vi "FestoCPX.Station.LaserPress.Ready.vi"(7 "Log (T)":bool=TRUE, 8 "error in":errorcluster, 10 "Position":T2) -> (0 "error out":errorcluster, 2 "Ready state":T1)   [LabVIEW 2015]
uses:
  tools/Translator/Translator.Message.ctl
  tools/EventLog/EventLog.EventSource.ctl
  FestoCPX.Station.LaserPress.ReadyState.ctl
  tools/EventLog/EventLog.CreateError(array).vi
  Station/Station.ValvePosition.ctl
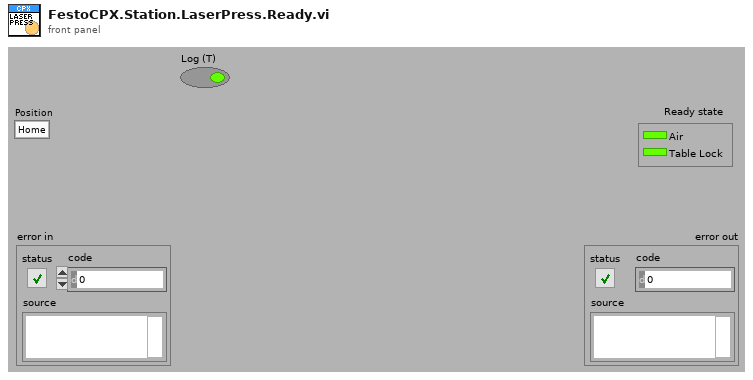
[diagram p1: front panel]
types:
  T1 = typedef "FestoCPX.Station.LaserPress.ReadyState.ctl" = cluster{"Air":bool, "Table Lock":bool}
  T2 = typedef "Station.ValvePosition.ctl" = enum16{"Home", "Work"}
  T3 = typedef "EventLog.EventSource.ctl" = enum16{"All", "Gui", "Ref", "File", "Seq", "Scan", "Lock", "AO", "AI", "CI", "DIO", "CPX", "PS", "Proda", "Trace", "Laser", "Keyence"}
  T4 = typedef "Translator.Message.ctl" = enum16{"-", "Event confirmed", "Log out", "Log in", "Shutdown", "Cancel", "Start", "On", "Off", "OK", "NOK", "NOK %s", "Home", "Work", "In progress...", "Missing", "Empty", "Hardware failure", "Initial", "Error %d >> %s", "Error %d >> %s >> %s", "Msg %d >> %s", "Unable to reset Laser Interlock", "Unable to reset Laser Shutterlock. Laser not ready", "Starting %s", "Quitting %s", "Configured", "Initializing", "Quitting", "Loading", "Running", "Stopped", "Summary", "Laser", "Do you want to continue?", "Station is not based. Do you want to exit?", "Station requires changeover. Do you want to run the test?", "Test options are not set as default. Do you want to continue?", "Connect ATEQ to terminal and set leakage to 0", "Set no leakage at ATEQ", "Set desired leakage at ATEQ at terminal M1 or skip", "Set desired leakage at ATEQ at terminal M3/M21/M22 or skip", "Set desired leakage at ATEQ at terminal M12 or skip", "Set desired leakage at ATEQ at terminal M1/M3 or skip", "Set desired leakage at ATEQ at terminal M21/M22 or skip", "Set desired leakage at ATEQ at terminal M1/M21/M22 or skip", "Calibration", "Log out?", "System", "All", "IDLE", "Translating...%s", "Not found", "Alarm %s", "Run", "Skip", "Abort", "Repeat", "Please wait...", "Database disconnected", "Database disconnected - changeover disabled!", "Login to database successful", "Login to database failed: %d; %s", "Unable to check the product status of reference %d - database disconnected", "Unable to set the product status of reference %d - database disconnected", "Variant file backup %s", "Read steps (%s)", "Result", "Station armed!", "Station requires changeover!", "Select reference number...", "EMERGENCY CURTAIN", "EMERGENCY BUTTON - press Control button", "EMERGENCY DOOR - press Control button", "Unable to reset safety circuit - Emergency Button pressed", "Unable to reset safety circuit - Emergency Doors open", "Station not based", "Station basing...", "Unkown reference", "Reference %d missing", "Test %s", "Test OK", "Test NOK", "Test NOK - press Confirm button", "Test error - press Confirm button", "Test stopped", "Station ready / Prepare product", "Station ready / Press start to scan product", "Station ready / Scanning product", "Rotating table...", "Rotating table... on hold by curtain", "Table rotated in %.1f seconds", "Table rotation aborted - Emergency button", "Table rotation aborted - Emergency door", "Table rotation aborted - Air pressure 1 off", "Table rotation aborted - Air pressure 2 off", "Test running... / Prepare next product", "Test running... / Press start to scan next product", "Test running... / Scanning next product...", "Test running... / Next products will start automatically", "Test running... / Scanning failed", "Stopping test...", "Finalizing test...", "Sequence folder '%s' is missing", "File '%s' is missing", "File '%s' is broken", "File '%s' is running", "Log file '%s' started", "Step '%s' added to log file", "Step '%s' graph added to log file", "Log file '%s' ended", "Log file '%s' ignored", "Log file '%s' exported", "Log file '%s' export failed", "Wrong serial number in log file", "Test steps are missing", "Output %s = %.3f", "Unable to output %s = %.1f (FB = %.1f; SP = %.1f)", "Unable to stabilize %s = %.1f (SP = %.1f)", "Assembly timeout", "Disassembly timeout", "Assembly %d | %25s | %.02f | %d", "Disassembly %d | %25s | %.02f | %d", "Process param '%s' not found in DB", "Process param '%s' wrong order", "Process param '%s' value %.3f out of limits (%.3f; %.3f)", "Step%d param '%s' not found in DB", "Step%d param '%s' wrong order", "Step%d param '%s' value %.3f out of limits (%.3f; %.3f)", "Step%d EV '%s' not found in DB", "Step%d EV '%s' wrong order", "Reference %d accepted", "Sequence started", "Sequence done", "Sequence aborted at step %d", "Sequence aborted at work", "Sequence aborted at home", "Sequence stopped at step %d", "Sequence error at step %d", "Seqeunce error at home", "Sequence error at work", "Scan plate failed", "Scan laser failed", "Scan plate failed. Error %s", "Scan laser failed. Error %s", "Scan plate failed. Scanner disconnected", "Scan laser failed. Scanner disconnected", "Scan plate failed. Wrong reference %d (expected %d)", "Scan plate failed. Serial number %d/%d did not pass the previous station (status %d)", "Scan plate OK %d/%d", "Scan laser OK", "Scan plate failed. Code missing", "Scan laser failed. Code missing", "Plate scanner OK", "Plate scanner failed. Press confirm button", "Scanning plate...", "%s = %d", "%s = %d->%d", "Motor initialized", "Motor homing", "Motor homed", "Motor home timeout", "Motor home failure. Unable to reset encoder counter (motor pos %.2f; enc pos %.2f)", "Motor started @ %.2f (%s; %.2f; %.1f)", "Motor updated @ %.2f (%s; %.2f; %.1f)", "Motor stopped @ %.2f", "Motor stop timeout", "Motor reached the position @ %.2f", "Motor reached the torque @ %.2f; %.2f", "Motor reached the pressure @ %.2f; %.2f", "Motor timeout (sp %.2f; pv %.2f)", "Unable to move motor - Forks not in Home position", "Screwdriver start timeout", "Screwdriver stop timeout", "Not homed", "Leak test timeout", "Unable to set %s = %.2f - air pressure off", "Unable to reset Emergency Circuit - emg button", "Unable to reset Emergency Circuit - light curtain", "Unable to reset Emergency Circuit - door open", "Unable to set digital output '%s' = %d", "Unable to switch on Air Main Valve - timeout", "Unable to switch off Air Main Valve - timeout", "Unable to rotate Table - timeout", "Unable to rotate Table - air pressure off", "Unable to rotate Table - Press not in Home position", "Unable to rotate Table - Pneumatic & Electric Conn not in Home position", "Unable to rotate Table - Exhaust Conn not in Home position", "Unable to rotate Table - unlock before movement timeout", "Unable to rotate Table - lock after movement timeout", "Unable to move Table Lock to %s position - timeout", "Unable to move Table Lock to %s position - air pressure off", "Unable to move Table Lock to %s position - Table not in position", "Unable to move Product Press to %s position - timeout", "Unable to move Product Press to %s position - air pressure off", "Unable to move Product Press to %s position - Table not locked", "Unable to move Product Press to %s position - Pneumatic & Electric Conn not in Home position", "Unable to move Product Press to %s position - Exhaust Conn not in Home position", "Unable to move Pneumatic & Electric Conn to %s position - timeout", "Unable to move Pneumatic & Electric Conn to %s position - air pressure off", "Unable to move Pneumatic & Electric Conn to %s position - Product Press not in Work position", "Unable to move Vent %s to %s position - timeout", "Unable to move Vent %s to %s position - air pressure off", "Unable to move Vent %s to %s position - Product Press not in Work position", "Unable to move Laser Press to %s position - timeout", "Unable to move Laser Press to %s position - air pressure off", "Unable to move Laser Press to %s position - Table not locked"}
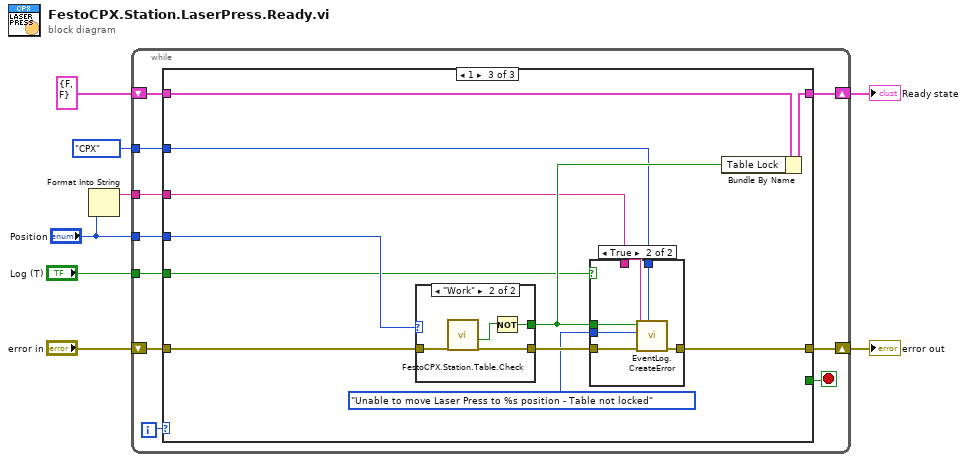
[diagram p0: block diagram]
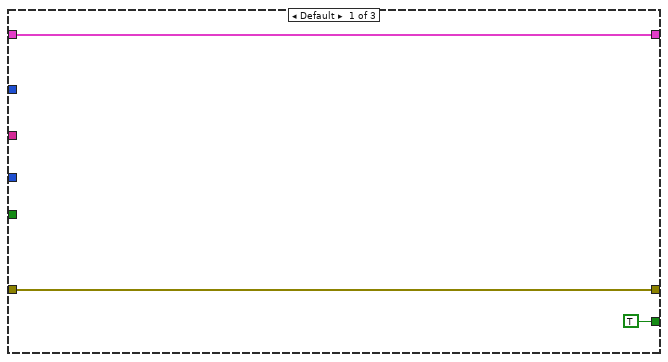
[diagram p2: hidden frame]
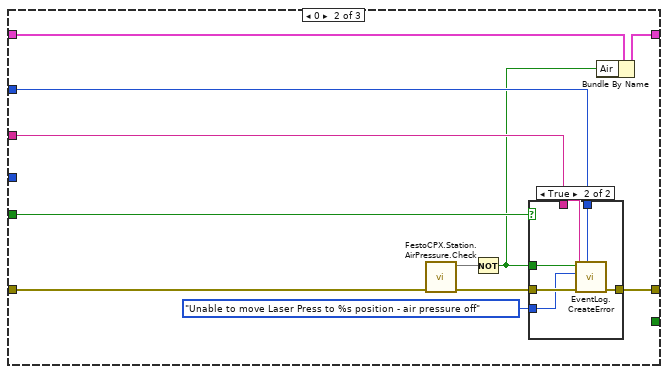
[diagram p3: hidden frame]
diagram:
  n1 = Format Into String("Position") -> (resulting string=w2:string)  [unwired: 3 in, 1 out]
  n2 = while {
    tunnel: "Log (T)" -> [w17]
    tunnel: w2 -> [w16]
    tunnel: EventLog.EventSource."CPX" ("Source") -> [w15]
    shift-right: [w10] -> w5
    shift-left: "error in" -> [w18]
    shift-right: [w11] -> w3
    shift-left: T1 {"Air"=FALSE, "Table Lock"=FALSE} ("Ready state") -> [w12]
    tunnel: "Position" -> [w9]
    i -> [w14]
    stop <- w13 stop-if-true
    n3 = case shown="1" w14 {
      tunnel: w18 -> [w20 w23 w42]
      tunnel: [w19 w26 w47] -> w11
      tunnel: w17 -> [_ w25 w43]
      tunnel: w16 -> [_ w29 w45]
      tunnel: w15 -> [_ w28 w46]
      tunnel: [TRUE _ _] -> w13
      tunnel: w12 -> [w19 w27 w48]
      tunnel: [w20 w30 w49] -> w10
      tunnel: w9 -> [_ _ w44]
      frame Default {
      }
      frame 0 {
        n4 = call "FestoCPX.Station.AirPressure.Check.vi"("error in"=w23) -> ("error out"=w32:errorcluster, 3:w24)  [unwired: 7 in, 2 out]
        n5 = Not(x=w24) -> (.not. x?=w22:bool)
        n6 = case shown="True" w25 {
          tunnel: w28 -> [_ w39]
          tunnel: w22 -> [_ w38]
          tunnel: w32 -> [w33 w37]
          tunnel: w29 -> [_ w36]
          tunnel: Translator.Message."Unable to move Laser Press to %s position - air pressure off" ("msg") -> [_ w35]
          tunnel: [w33 w34] -> w30
          frame False {
          }
          frame True {
            n7 = call-poly "EventLog.CreateError.vi"("Source (All)"=w39, "error in"=w37, "args"=w36, "msg"=w35, "create (T)"=w38) -> ("error out"=w34:errorcluster)  [unwired: 5 in, 1 out]
          }
        }
        n8 = Bundle By Name(cluster=w27, "Air"=w22) -> (w26:T1)
      }
      frame 1 {
        n9 = case shown="\"Work\"" w44 {
          tunnel: w42 -> [w51 w55]
          tunnel: [w51 w54] -> w41
          tunnel: [_ w53] -> w50
          frame "Home" {
          }
          frame "Work" {
            n10 = call "FestoCPX.Station.Table.Check.vi"("error in"=w55) -> ("error out"=w54:errorcluster, "Table Lock"=w52:bool)  [unwired: 8 in, 1 out]
            n11 = Not(x=w52) -> (.not. x?=w53:bool)
          }
        }
        n12 = case shown="True" w43 {
          tunnel: w46 -> [_ w62]
          tunnel: w50 -> [_ w61]
          tunnel: w41 -> [w56 w60]
          tunnel: w45 -> [_ w59]
          tunnel: Translator.Message."Unable to move Laser Press to %s position - Table not locked" ("msg") -> [_ w58]
          tunnel: [w56 w57] -> w49
          frame False {
          }
          frame True {
            n13 = call-poly "EventLog.CreateError.vi"("Source (All)"=w62, "error in"=w60, "args"=w59, "msg"=w58, "create (T)"=w61) -> ("error out"=w57:errorcluster)  [unwired: 5 in, 1 out]
          }
        }
        n14 = Bundle By Name(cluster=w48, "Table Lock"=w50) -> (w47:T1)
      }
    }
  }
  "error out" <- w5
  "Ready state" <- w3
